vi "Main.vi"() -> ()   [LabVIEW 2018]
uses:
  Controls/Sys or Set Clock.ctl
  Controls/Time.ctl
  Controls/Set or Cancel Alarm.ctl
  Controls/Alarm Mode.ctl
  Controls/Show Stopwatch.ctl
panel:
  out "Stopwatch Value(ms)":ext format="%#.0f"
  in  "Reset Stopwatch":bool
  in  "Start/Pause Stopwatch":bool
  in  "Show Stopwatch":T1
  out "Clock Numbers":picture
  in  "Alarm Photo Path":path
  out "Alarm Photo":picture
  in  "Alarm Mode":T2 items=["Sound Mode", "Photo Mode"]
  in  "Alarm Sound Path":path
  out "isAlarmSet":bool
  in  "Alarm Minute":i32(slide) min=0 max=59 step=1 scale=0.0..59.0
  in  "Alarm Hour":i32(slide) min=0 max=23 step=1 scale=0.0..23.0
  in  "Set/Cancel Alarm":T3
  out "Time":T4
  in  "Set  Hour":i32(knob) scale=0.0..24.0
  in  "Set  Minute":i32(knob) scale=0.0..60.0
  in  "Set Second":i32(knob) scale=0.0..60.0
  in  "Sys/Set Clock":T5
  out "AM/PM":string
  out "Clock":cluster{dbl[], dbl[]}[](graph)=[{array[628 elements], array[628 elements]}, {[0.0, 2.041077998578922e-17, 4.082155997157844e-17], [0.0, 0.3333333333333333, 0.6666666666666666]}, {[0.0, 3.061616997868383e-17], [0.0, 0.5]}, {array[628 elements], array[628 elements]}] caption="XY Graph"
  in  "stop":bool
  out "pi/180":dbl
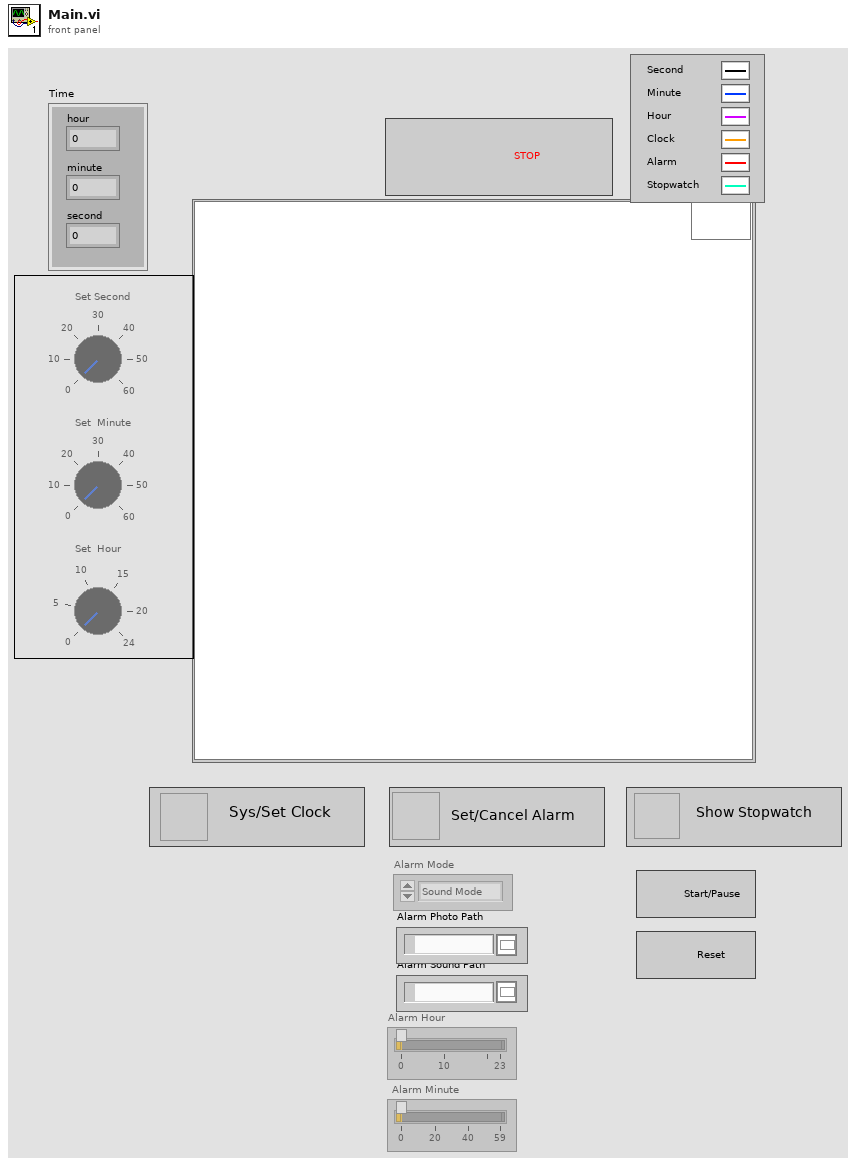
[diagram p1: front panel]
types:
  T1 = typedef "Show Stopwatch.ctl" = bool
  T2 = typedef "Alarm Mode.ctl" = u16
  T3 = typedef "Set or Cancel Alarm.ctl" = bool
  T4 = typedef "TIme.ctl" = cluster{"hour":i32, "minute":i32, "second":i32}
  T5 = typedef "Sys or Set Clock.ctl" = bool
  T6 = enum8{"Enabled", "Disabled", "Disabled and Grayed Out"}
  T7 = typedef "LVDateTimeRec.ctl" = cluster{"fractional second":dbl, "second":i32, "minute":i32, "hour":i32, "day of month":i32, "month":i32, "year":i32, "day of week":i32, "day of year":i32, "DST":i32}
  T8 = typedef "Sound Output Task ID.ctl" = u32
  T9 = typedef "imagedata.ctl" = cluster{"image type":i32, "image depth":i32, "image":u8[], "mask":u8[], "colors":u32[], "Rectangle":cluster{"left":i16, "top":i16, "right":i16, "bottom":i16}}
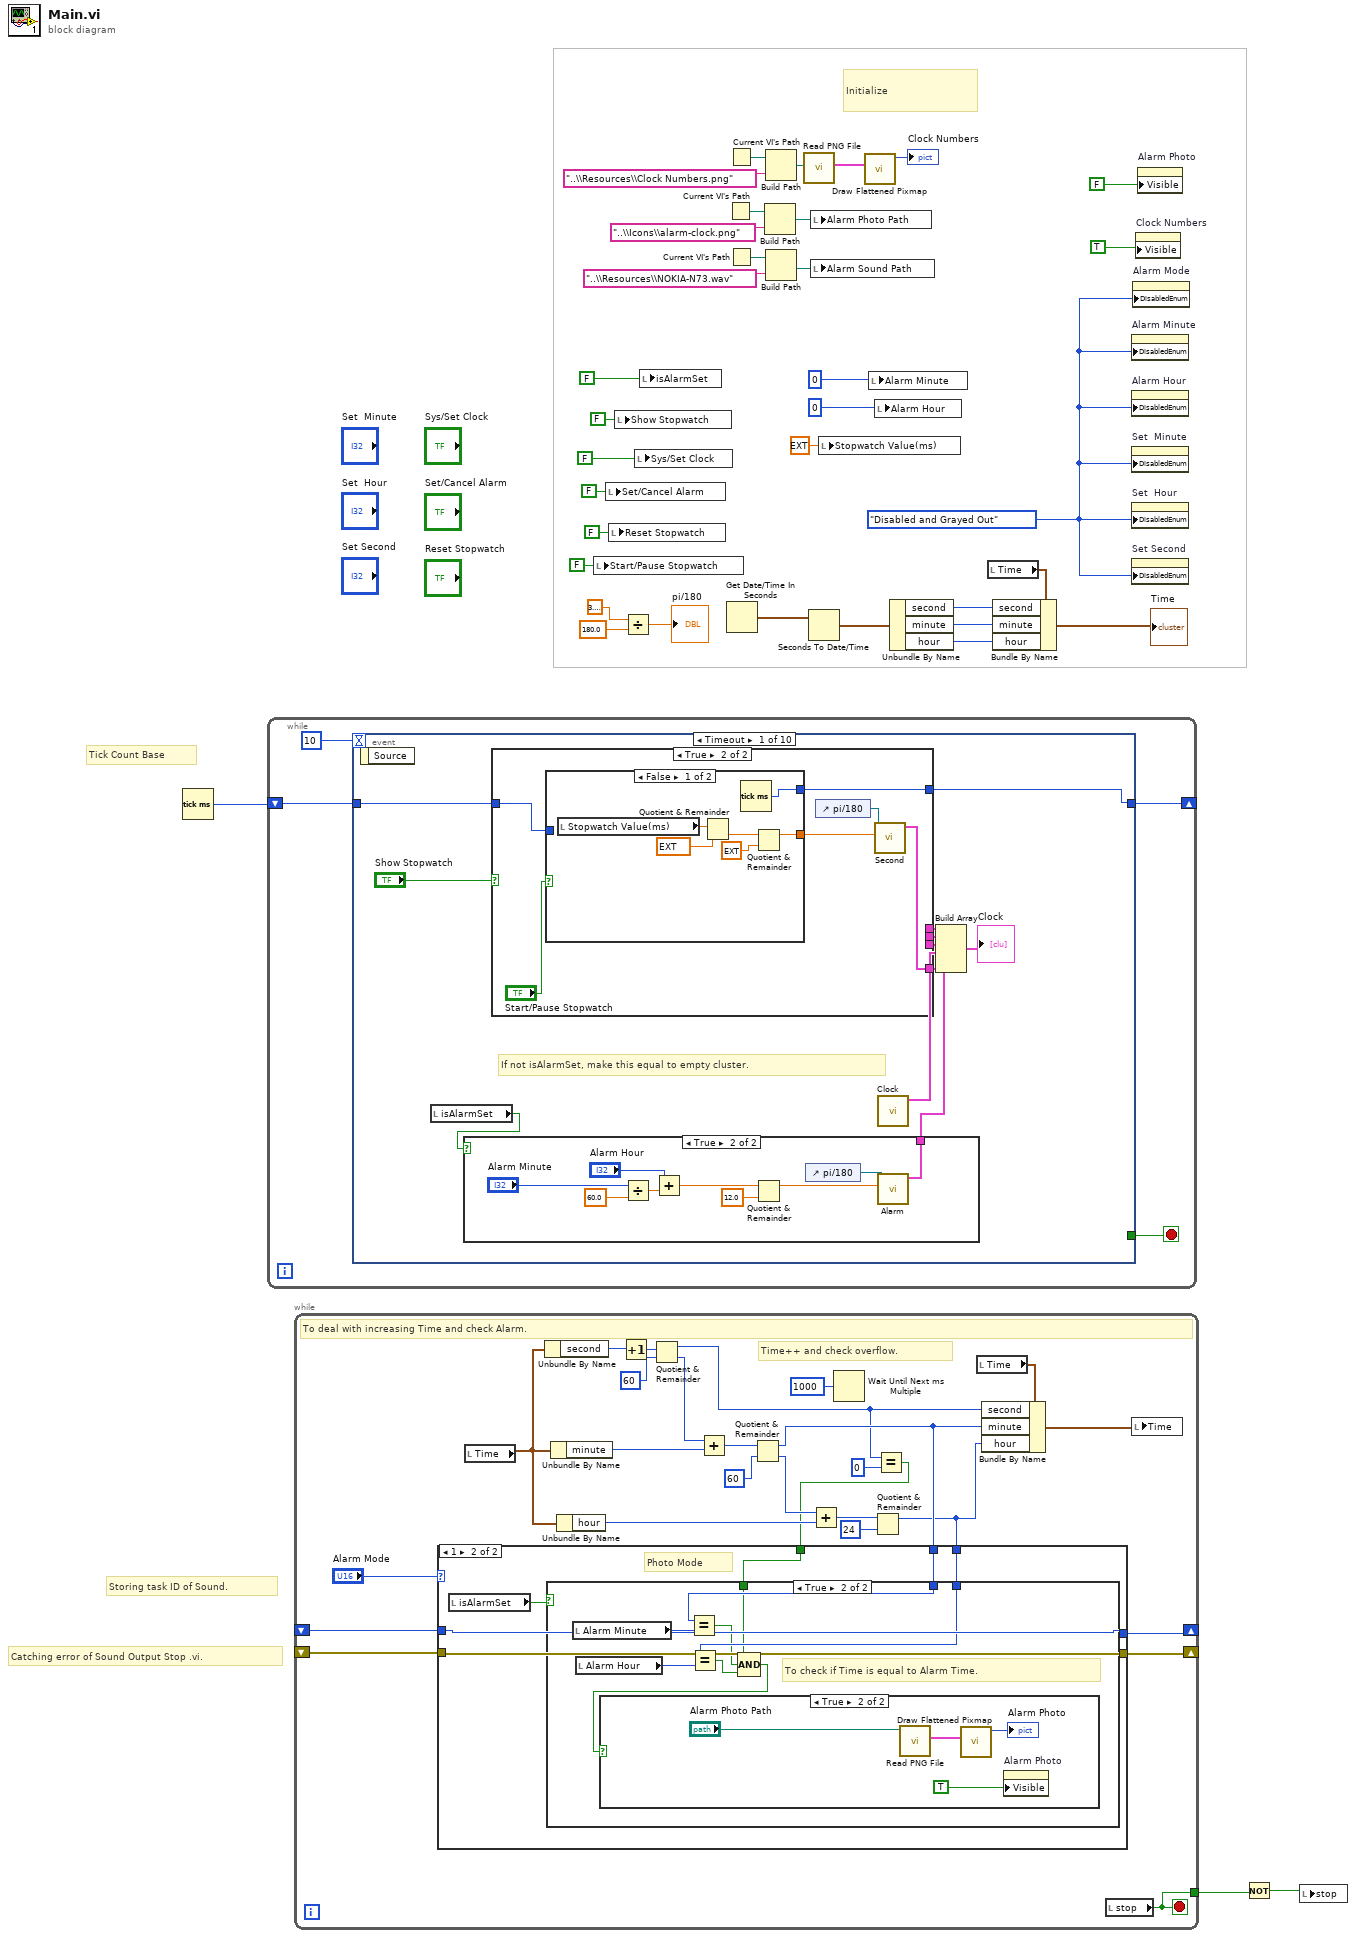
[diagram p0: block diagram]
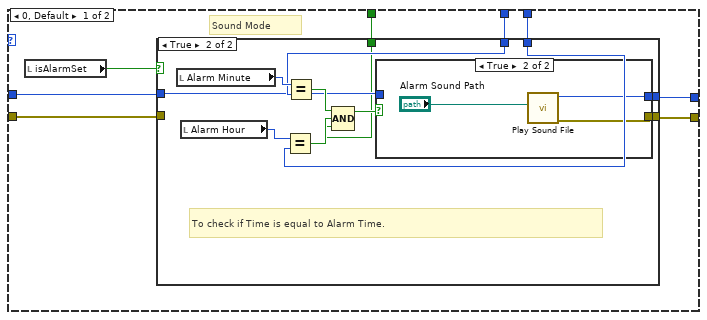
[diagram p2: hidden frame]
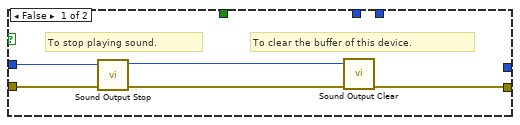
[diagram p3: hidden frame]
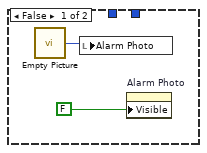
[diagram p5: hidden frame]
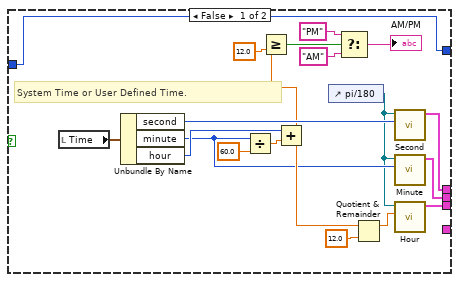
[diagram p7: hidden frame]
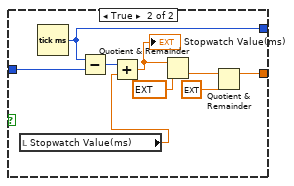
[diagram p8: hidden frame]
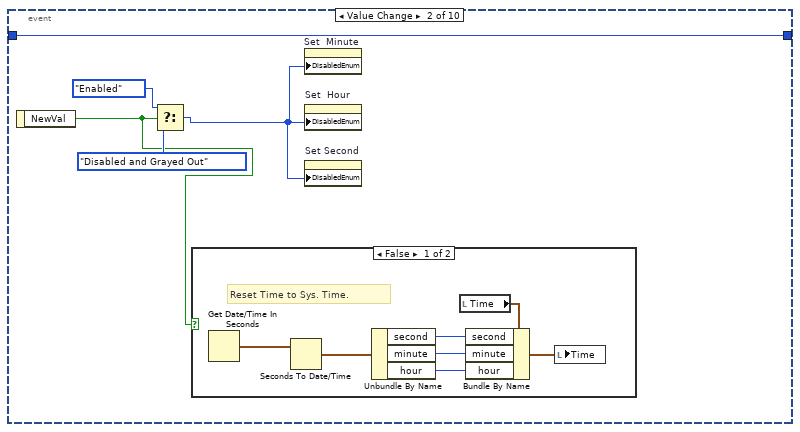
[diagram p10: hidden frame]
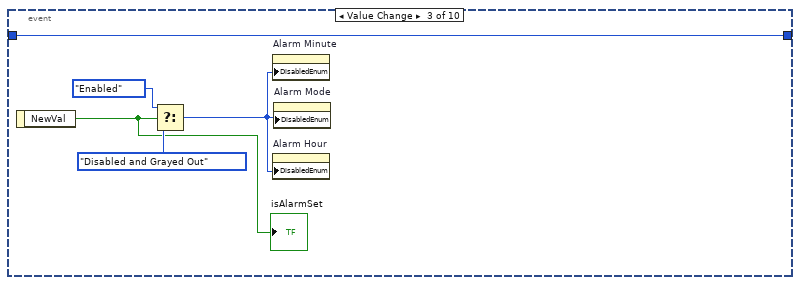
[diagram p12: hidden frame]
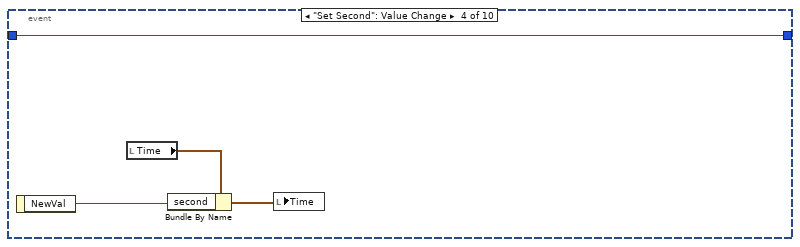
[diagram p13: hidden frame]
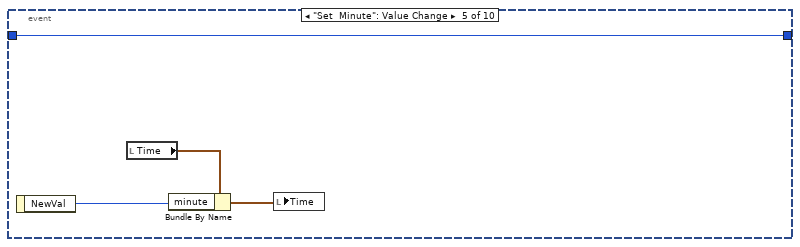
[diagram p14: hidden frame]
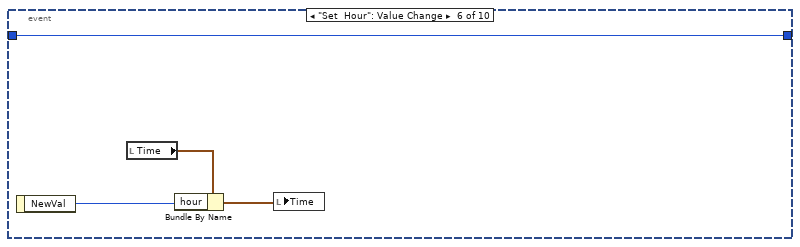
[diagram p15: hidden frame]
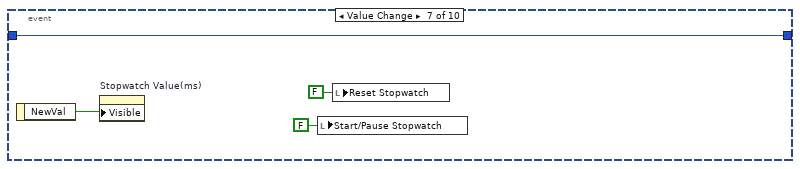
[diagram p16: hidden frame]
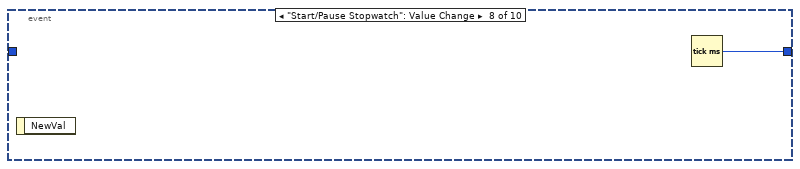
[diagram p17: hidden frame]
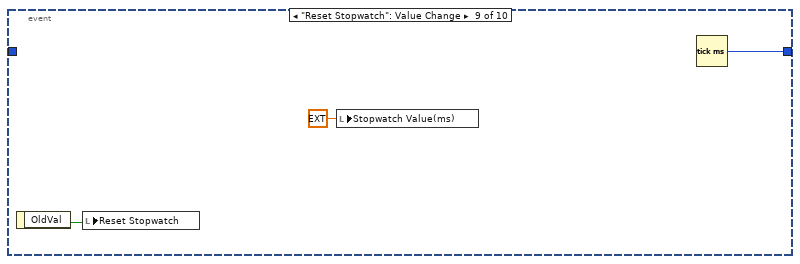
[diagram p18: hidden frame]
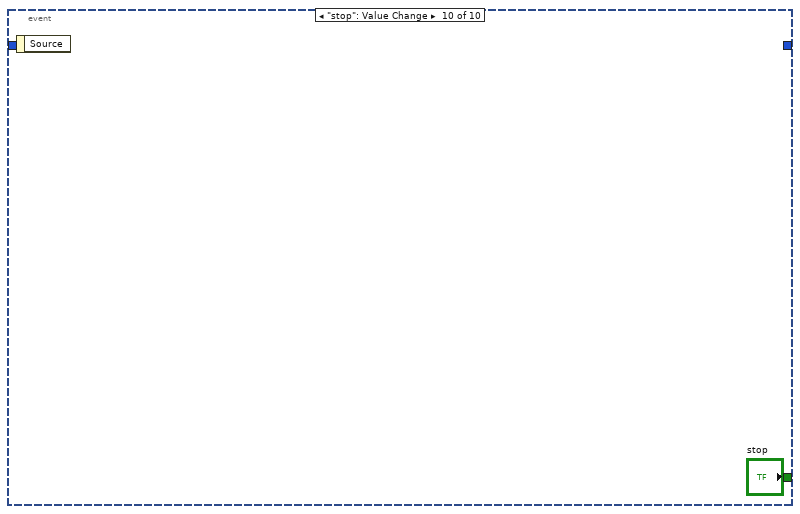
[diagram p19: hidden frame]
diagram:
  w13 = T6."Disabled and Grayed Out" ("Disabled")
  # "Tick Count Base"
  # "Catching error of Sound Output Stop .vi."
  # "Storing task ID of Sound."
  # "Initialize"
  n1 = Tick Count (ms)() -> (millisecond timer value=w6:u32)
  n2 = while {
    shift-right: [w37] -> _
    shift-left: w6 -> [w38]
    stop <- w39 stop-if-true
    n3 = event shown="[0] Timeout" {
      selector: _ -> [_ _ _ _ _ _ _ _ _ _]
      dyn-events: _ -> [_ _ _ _ _ _ _ _ _ _]
      timeout: 10 -> [_ _ _ _ _ _ _ _ _ _]
      tunnel: [_ _ _ _ _ _ _ _ _ "stop"] -> w39
      tunnel: w38 -> [w42 w101 w113 w118 w122 w126 w132 _ _ _]
      tunnel: [w41 w101 w113 w118 w122 w126 w132 w134 w137 _] -> w37
      event Timeout {
        # "If not isAlarmSet, make this equal to empty cluster."
        n4 = event-data() -> ()  [unwired: 1 in, 1 out]
        n5 = local read "isAlarmSet"() -> (w46:bool)
        n6 = case shown="True" w46 {
          tunnel: [_ w93] -> w45
          frame False {
          }
          frame True {
            n7 = Divide(x="Alarm Minute", y=60.0) -> (x/y=w98:dbl)
            n8 = Add(x="Alarm Hour", y=w98) -> (x+y=w100:dbl)
            n9 = Quotient & Remainder(x=w100, y=12.0) -> (x-y*floor(x/y)=w94:dbl)  [unwired: 1 out]
            n10 = control-ref of="pi/180"() -> (w92:refnum<vi>)
            n11 = call "Alarm.vi"("Numeric"=w94, "Digital in"=w92) -> ("Cluster"=w93:cluster{dbl[], dbl[]})  [unwired: 9 in]
          }
        }
        n12 = case shown="True" "Show Stopwatch" {
          tunnel: [w61 _] -> w51
          tunnel: [w60 _] -> w50
          tunnel: [w59 _] -> w49
          tunnel: w42 -> [w52 w76]
          tunnel: [_ w75] -> w43
          tunnel: [w52 w71] -> w41
          frame False {
            # "System Time or User Defined Time."
            n13 = local read "Time"() -> (w58:T4)
            n14 = Unbundle By Name(w58) -> ("second"=w68:i32, "minute"=w56:i32, "hour"=w67:i32)
            n15 = Divide(x=w56, y=60.0) -> (x/y=w54:dbl)
            n16 = Add(x=w67, y=w54) -> (x+y=w57:dbl)
            n17 = Greater Or Equal?(x=w57, y=12.0) -> (x >= y?=w65:bool)
            n18 = control-ref of="pi/180"() -> (w53:refnum<vi>)
            n19 = Select(t="PM", s=w65, f="AM") -> (s? t:f=→"AM/PM":string)
            n20 = Quotient & Remainder(x=w57, y=12.0) -> (x-y*floor(x/y)=w70:dbl)  [unwired: 1 out]
            n21 = call "Second.vi"("second"=w68, "Digital in"=w53) -> ("Cluster"=w61:cluster{dbl[], dbl[]})  [unwired: 9 in]
            n22 = call "Minute.vi"("minute"=w56, "Digital in"=w53) -> ("Cluster"=w60:cluster{dbl[], dbl[]})  [unwired: 9 in]
            n23 = call "Hour.vi"("Numeric"=w70, "Digital in"=w53) -> ("Cluster"=w59:cluster{dbl[], dbl[]})  [unwired: 9 in]
          }
          frame True {
            n24 = case shown="False" "Start/Pause Stopwatch" {
              tunnel: w76 -> [_ w91]
              tunnel: [w78 w87] -> w74
              tunnel: [w77 w83] -> w71
              frame False {
                n25 = local read "Stopwatch Value(ms)"() -> (w80:ext)
                n26 = Quotient & Remainder(x=w80, y=ext 1000.0) -> (floor(x/y)=w82:ext)  [unwired: 1 out]
                n27 = Tick Count (ms)() -> (millisecond timer value=w77:u32)
                n28 = Quotient & Remainder(x=w82, y=ext 60.0) -> (x-y*floor(x/y)=w78:ext)  [unwired: 1 out]
              }
              frame True {
                n29 = local read "Stopwatch Value(ms)"() -> (w85:ext)
                n30 = Tick Count (ms)() -> (millisecond timer value=w83:u32)
                n31 = Subtract(x=w83, y=w91) -> (x-y=w86:u32)
                n32 = Add(x=w86, y=w85) -> (x+y=w84:ext)
                "Stopwatch Value(ms)" <- w84
                n33 = Quotient & Remainder(x=w84, y=ext 1000.0) -> (floor(x/y)=w89:ext)  [unwired: 1 out]
                n34 = Quotient & Remainder(x=w89, y=ext 60.0) -> (x-y*floor(x/y)=w87:ext)  [unwired: 1 out]
              }
            }
            n35 = control-ref of="pi/180"() -> (w72:refnum<vi>)
            n36 = call "Second.vi"("second"=w74, "Digital in"=w72) -> ("Cluster"=w75:cluster{dbl[], dbl[]})  [unwired: 9 in]
          }
        }
        n37 = call "Clock.vi"() -> ("Cluster"=w47:cluster{dbl[], dbl[]})  [unwired: 11 in]
        n38 = Build Array(w51, w50, w49, w47, w45, w43) -> (→"Clock":cluster{dbl[], dbl[]}[])
      }
      event Value Change {
        n39 = event-data() -> ("NewVal"=w102:T5)  [unwired: 1 in]
        n40 = Select(t=T6."Enabled" ("Disabled"), s=w102, f=T6."Disabled and Grayed Out" ("Disabled")) -> (s? t:f=w104:T6)
        n41 = case shown="False" w102 {
          frame False {
            # "Reset Time to Sys. Time."
            n42 = Get Date/Time In Seconds() -> (seconds since 1Jan1904=w108:timestamp)
            n43 = Seconds To Date/Time(time stamp (now)=w108) -> (date time rec=w109:T7)  [unwired: 1 in]
            n44 = Unbundle By Name(w109) -> ("second"=w110:i32, "minute"=w111:i32, "hour"=w112:i32)
            n45 = local read "Time"() -> (w107:T4)
            n46 = Bundle By Name(cluster=w107, "second"=w110, "minute"=w111, "hour"=w112) -> (w106:T4)
            n47 = local write "Time"(w106) -> ()
          }
          frame True {
          }
        }
        n48 = property on="Set  Minute" class="Knob (strict)"("DisabledEnum"=w104) -> ()  [unwired: 2 in, 2 out]
        n49 = property on="Set  Hour" class="Knob (strict)"("DisabledEnum"=w104) -> ()  [unwired: 2 in, 2 out]
        n50 = property on="Set Second" class="Knob (strict)"("DisabledEnum"=w104) -> ()  [unwired: 2 in, 2 out]
      }
      event Value Change {
        n51 = event-data() -> ("NewVal"=w115:T3)  [unwired: 1 in]
        "isAlarmSet" <- w115
        n52 = Select(t=T6."Enabled" ("Disabled"), s=w115, f=T6."Disabled and Grayed Out" ("Disabled")) -> (s? t:f=w114:T6)
        n53 = property on="Alarm Minute" class="Slide (strict)"("DisabledEnum"=w114) -> ()  [unwired: 2 in, 2 out]
        n54 = property on="Alarm Hour" class="Slide (strict)"("DisabledEnum"=w114) -> ()  [unwired: 2 in, 2 out]
        n55 = property on="Alarm Mode" class="Ring (strict)"("DisabledEnum"=w114) -> ()  [unwired: 2 in, 2 out]
      }
      event "Set Second": Value Change {
        n56 = event-data() -> ("NewVal"=w121:i32)  [unwired: 1 in]
        n57 = local read "Time"() -> (w120:T4)
        n58 = Bundle By Name(cluster=w120, "second"=w121) -> (w119:T4)
        n59 = local write "Time"(w119) -> ()
      }
      event "Set  Minute": Value Change {
        n60 = event-data() -> ("NewVal"=w125:i32)  [unwired: 1 in]
        n61 = local read "Time"() -> (w124:T4)
        n62 = Bundle By Name(cluster=w124, "minute"=w125) -> (w123:T4)
        n63 = local write "Time"(w123) -> ()
      }
      event "Set  Hour": Value Change {
        n64 = event-data() -> ("NewVal"=w129:i32)  [unwired: 1 in]
        n65 = local read "Time"() -> (w128:T4)
        n66 = Bundle By Name(cluster=w128, "hour"=w129) -> (w127:T4)
        n67 = local write "Time"(w127) -> ()
      }
      event Value Change {
        n68 = event-data() -> ("NewVal"=w133:T1)  [unwired: 1 in]
        n69 = property on="Stopwatch Value(ms)" class="DigNum (strict)"("Visible"=w133) -> ()  [unwired: 2 in, 2 out]
        n70 = local write "Start/Pause Stopwatch"(FALSE ("Start/Pause Stopwatch")) -> ()
        n71 = local write "Reset Stopwatch"(FALSE ("Reset Stopwatch")) -> ()
      }
      event "Start/Pause Stopwatch": Value Change {
        n72 = event-data() -> ()  [unwired: 1 in, 1 out]
        n73 = Tick Count (ms)() -> (millisecond timer value=w134:u32)
      }
      event "Reset Stopwatch": Value Change {
        n74 = event-data() -> ("OldVal"=w135:bool)  [unwired: 1 in]
        n75 = local write "Reset Stopwatch"(w135) -> ()
        n76 = local write "Stopwatch Value(ms)"(ext 0.0 ("Stopwatch Value(ms)")) -> ()
        n77 = Tick Count (ms)() -> (millisecond timer value=w137:u32)
      }
      event "stop": Value Change {
        n78 = event-data() -> ()  [unwired: 1 in, 1 out]
      }
    }
  }
  n79 = while {
    tunnel: [w149] -> w26
    shift-right: [w146] -> _
    shift-left: _ -> [w145]
    shift-right: [w144] -> _
    shift-left: _ -> [w143]
    stop <- w149 stop-if-true
    # "Time++ and check overflow."
    # "To deal with increasing Time and check Alarm."
    n80 = local read "Time"() -> (w157:T4)
    n81 = Unbundle By Name(w157) -> ("second"=w164:i32)
    n82 = Unbundle By Name(w157) -> ("minute"=w161:i32)
    n83 = Unbundle By Name(w157) -> ("hour"=w156:i32)
    n84 = Increment(x=w164) -> (x+1=w163:i32)
    n85 = Quotient & Remainder(x=w163, y=60) -> (x-y*floor(x/y)=w142:i32, floor(x/y)=w160:i32)
    n86 = Add(x=w160, y=w161) -> (x+y=w159:i32)
    n87 = Quotient & Remainder(x=w159, y=60) -> (x-y*floor(x/y)=w148:i32, floor(x/y)=w155:i32)
    n88 = Add(x=w155, y=w156) -> (x+y=w154:i32)
    n89 = Wait Until Next ms Multiple(millisecond multiple=u32 1000 ("milliseconds to wait")) -> ()  [unwired: 1 out]
    n90 = Quotient & Remainder(x=w154, y=24) -> (x-y*floor(x/y)=w147:i32)  [unwired: 1 out]
    n91 = Equal?(x=w142, y=0) -> (x = y?=w140:bool)
    n92 = case shown="1" "Alarm Mode" {
      tunnel: w148 -> [w172 w195]
      tunnel: w147 -> [w171 w194]
      tunnel: [w170 w198] -> w146
      tunnel: w145 -> [w169 w198]
      tunnel: [w168 w197] -> w144
      tunnel: w143 -> [w167 w197]
      tunnel: w140 -> [w166 w193]
      frame 0, Default {
        # "Sound Mode"
        n93 = local read "isAlarmSet"() -> (w165:bool)
        n94 = case shown="True" w165 {
          tunnel: w172 -> [_ w187]
          tunnel: w171 -> [_ w185]
          tunnel: [_ w181] -> w170
          tunnel: w169 -> [w177 w179]
          tunnel: [w173 w180] -> w168
          tunnel: w167 -> [w176 _]
          tunnel: w166 -> [_ w178]
          frame False {
            # "To clear the buffer of this device."
            # "To stop playing sound."
            n95 = call <vilib>:"Sound Output Stop.vi"("error in (no error)"=w176, "task ID"=w177) -> ("error out"=w174:errorcluster, "task ID out"=w175:T8)  [unwired: 8 in]
            n96 = call <vilib>:"Sound Output Clear.vi"("error in (no error)"=w174, "task ID"=w175) -> ("error out"=w173:errorcluster)  [unwired: 9 in]
          }
          frame True {
            # "To check if Time is equal to Alarm Time."
            n97 = local read "Alarm Minute"() -> (w188:i32)
            n98 = local read "Alarm Hour"() -> (w186:i32)
            n99 = Equal?(x=w186, y=w185) -> (x = y?=w183:bool)
            n100 = Equal?(x=w188, y=w187) -> (x = y?=w184:bool)
            n101 = Compound Arithmetic op=AND(w184, w183, w178) -> (w182:bool)
            n102 = case shown="True" w182 {
              tunnel: [w189 w191] -> w181
              tunnel: [_ w190] -> w180
              tunnel: w179 -> [w189 _]
              frame False {
              }
              frame True {
                n103 = call <vilib>:"Play Sound File.vi"("path"="Alarm Sound Path") -> ("error out"=w190:errorcluster, "task ID"=w191:T8)  [unwired: 9 in]
              }
            }
          }
        }
      }
      frame 1 {
        # "Photo Mode"
        n104 = local read "isAlarmSet"() -> (w196:bool)
        n105 = case shown="True" w196 {
          tunnel: w195 -> [_ w207]
          tunnel: w194 -> [_ w206]
          tunnel: w193 -> [_ w204]
          frame False {
            n106 = call "Empty Picture"() -> ("empty picture"=w199:picture)
            n107 = local write "Alarm Photo"(w199) -> ()
            n108 = property on="Alarm Photo" class="Pict"("Visible"=FALSE) -> ()  [unwired: 2 in, 2 out]
          }
          frame True {
            # "To check if Time is equal to Alarm Time."
            n109 = local read "Alarm Minute"() -> (w208:i32)
            n110 = local read "Alarm Hour"() -> (w205:i32)
            n111 = Equal?(x=w207, y=w208) -> (x = y?=w203:bool)
            n112 = Equal?(x=w206, y=w205) -> (x = y?=w202:bool)
            n113 = Compound Arithmetic op=AND(w204, w203, w202) -> (w201:bool)
            n114 = case shown="True" w201 {
              frame False {
              }
              frame True {
                n115 = call <vilib>:"Read PNG File.vi"("path to PNG file"="Alarm Photo Path") -> ("image data"=w212:T9)  [unwired: 8 in, 2 out]
                n116 = call <vilib>:"Draw Flattened Pixmap.vi"("image data"=w212) -> ("new picture"=→"Alarm Photo":picture)  [unwired: 8 in]
                n117 = property on="Alarm Photo" class="Pict"("Visible"=TRUE) -> ()  [unwired: 2 in, 2 out]
              }
            }
          }
        }
      }
    }
    n118 = local read "Time"() -> (w152:T4)
    n119 = Bundle By Name(cluster=w152, "second"=w142, "minute"=w148, "hour"=w147) -> (w151:T4)
    n120 = local read "stop"() -> (w149:bool)
    n121 = local write "Time"(w151) -> ()
  }
  n122 = local write "Start/Pause Stopwatch"(FALSE ("Start/Pause Stopwatch")) -> ()
  n123 = local write "Set/Cancel Alarm"(T3 FALSE ("Set/Cancel Alarm")) -> ()
  n124 = local write "Reset Stopwatch"(FALSE ("Reset Stopwatch")) -> ()
  n125 = local write "Show Stopwatch"(T1 FALSE ("Show Stopwatch")) -> ()
  n126 = Divide(x=3.141592653589793, y=180.0) -> (x/y=→"pi/180":dbl)
  n127 = local write "Sys/Set Clock"(T5 FALSE ("Sys/Set Clock")) -> ()
  n128 = local write "isAlarmSet"(FALSE ("isAlarmSet")) -> ()
  n129 = Current VI's Path() -> (path=w15:path)
  n130 = Current VI's Path() -> (path=w11:path)
  n131 = Current VI's Path() -> (path=w22:path)
  n132 = Get Date/Time In Seconds() -> (seconds since 1Jan1904=w33:timestamp)
  n133 = Build Path(base path=w15, name or relative path="..\\Icons\\alarm-clock.png") -> (appended path=w14:path)
  n134 = Build Path(base path=w11, name or relative path="..\\Resources\\Clock Numbers.png") -> (appended path=w9:path)
  n135 = Build Path(base path=w22, name or relative path="..\\Resources\\NOKIA-N73.wav") -> (appended path=w21:path)
  n136 = call <vilib>:"Read PNG File.vi"("path to PNG file"=w9) -> ("image data"=w12:T9)  [unwired: 8 in, 2 out]
  n137 = Seconds To Date/Time(time stamp (now)=w33) -> (date time rec=w32:T7)  [unwired: 1 in]
  n138 = local write "Alarm Photo Path"(w14) -> ()
  n139 = local write "Alarm Sound Path"(w21) -> ()
  n140 = local write "Stopwatch Value(ms)"(ext 0.0 ("Stopwatch Value(ms)")) -> ()
  n141 = call <vilib>:"Draw Flattened Pixmap.vi"("image data"=w12) -> ("new picture"=→"Clock Numbers":picture)  [unwired: 8 in]
  n142 = local write "Alarm Minute"(0 ("Alarm Hour")) -> ()
  n143 = local write "Alarm Hour"(0 ("Alarm Hour")) -> ()
  n144 = Unbundle By Name(w32) -> ("second"=w30:i32, "minute"=w29:i32, "hour"=w28:i32)
  n145 = local read "Time"() -> (w31:T4)
  n146 = Bundle By Name(cluster=w31, "second"=w30, "minute"=w29, "hour"=w28) -> (→"Time":T4)
  n147 = property on="Alarm Minute" class="Slide (strict)"("DisabledEnum"=w13) -> ()  [unwired: 2 in, 2 out]
  n148 = property on="Alarm Hour" class="Slide (strict)"("DisabledEnum"=w13) -> ()  [unwired: 2 in, 2 out]
  n149 = property on="Set  Minute" class="Knob (strict)"("DisabledEnum"=w13) -> ()  [unwired: 2 in, 2 out]
  n150 = property on="Set  Hour" class="Knob (strict)"("DisabledEnum"=w13) -> ()  [unwired: 2 in, 2 out]
  n151 = property on="Set Second" class="Knob (strict)"("DisabledEnum"=w13) -> ()  [unwired: 2 in, 2 out]
  n152 = property on="Alarm Mode" class="Ring (strict)"("DisabledEnum"=w13) -> ()  [unwired: 2 in, 2 out]
  n153 = property on="Clock Numbers" class="Pict"("Visible"=TRUE) -> ()  [unwired: 2 in, 2 out]
  n154 = property on="Alarm Photo" class="Pict"("Visible"=FALSE) -> ()  [unwired: 2 in, 2 out]
  n155 = Not(x=w26) -> (.not. x?=w25:bool)
  n156 = local write "stop"(w25) -> ()
